vi "Translate.vi"(7 "Size":i32, 9 "direction in":enum16{"R", "D", "L", "U"}(ring), 10 "x in":i32, 11 "y in":i32) -> (1 "direction out":enum16{"R", "D", "L", "U"}(ring), 2 "x out":i32, 3 "y out":i32)   [LabVIEW 2021, in "d22.lvlib"]
uses:
  d22.lvlib
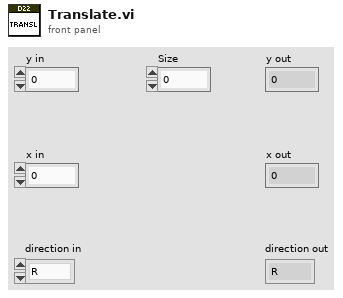
[diagram p1: front panel]
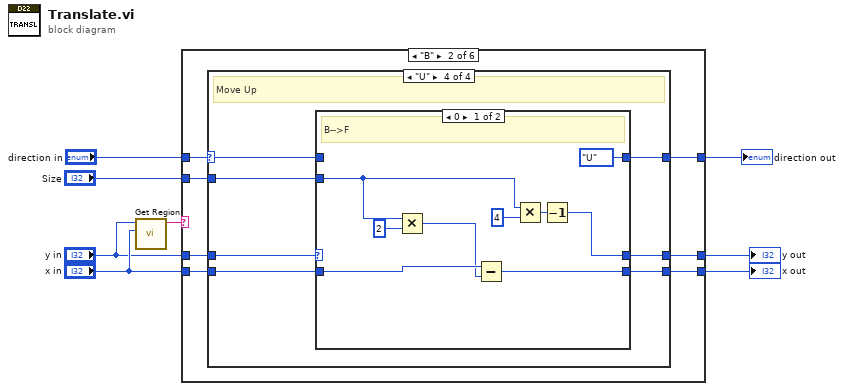
[diagram p0: block diagram]
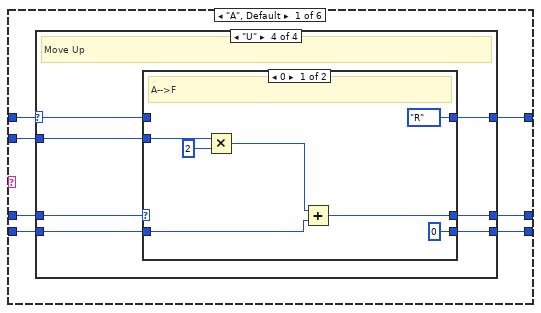
[diagram p2: hidden frame]
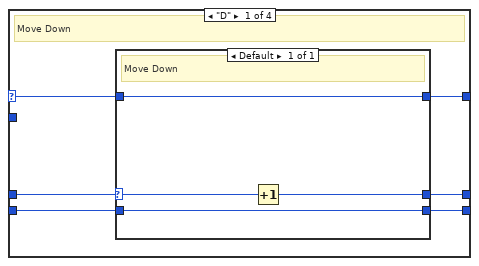
[diagram p3: hidden frame]
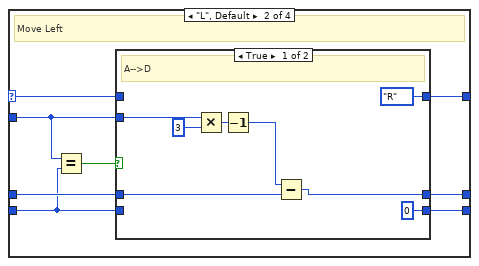
[diagram p4: hidden frame]
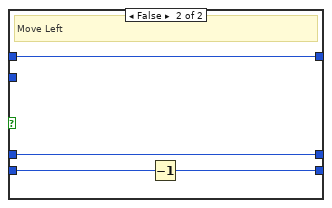
[diagram p5: hidden frame]
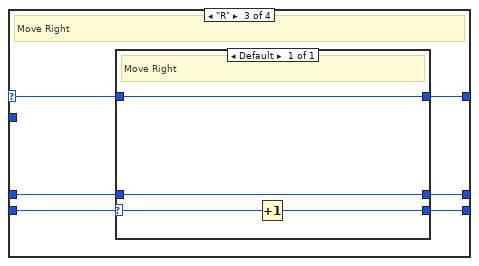
[diagram p6: hidden frame]
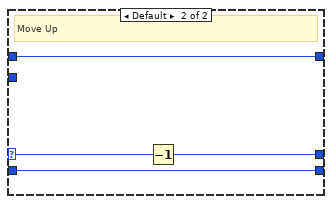
[diagram p7: hidden frame]
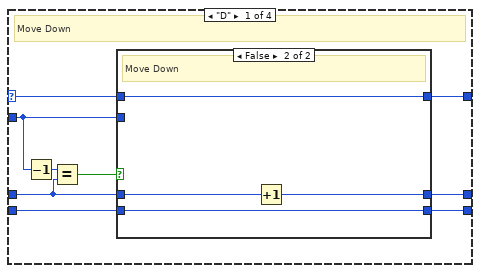
[diagram p8: hidden frame]
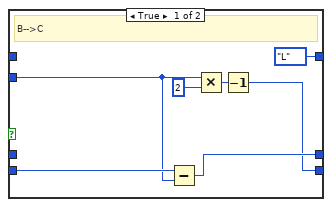
[diagram p9: hidden frame]
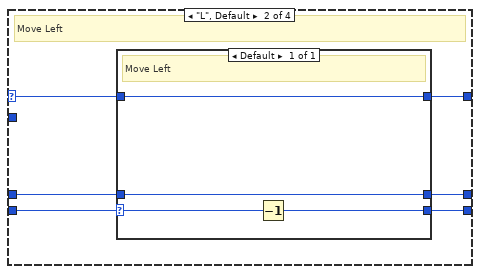
[diagram p10: hidden frame]
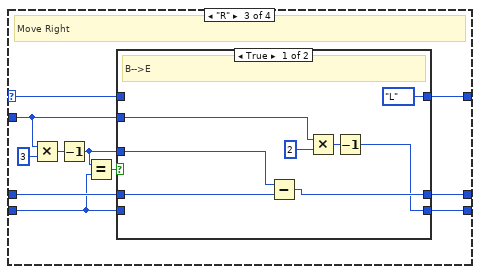
[diagram p11: hidden frame]
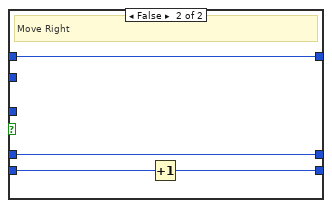
[diagram p12: hidden frame]
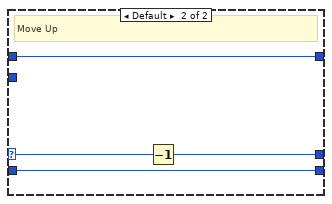
[diagram p13: hidden frame]
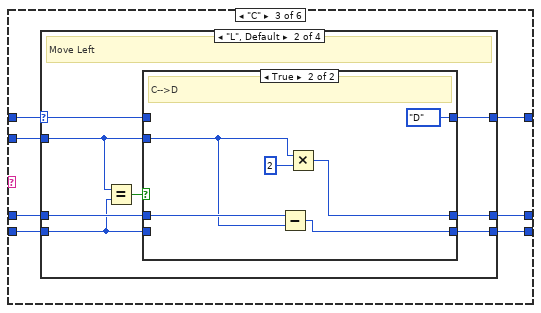
[diagram p14: hidden frame]
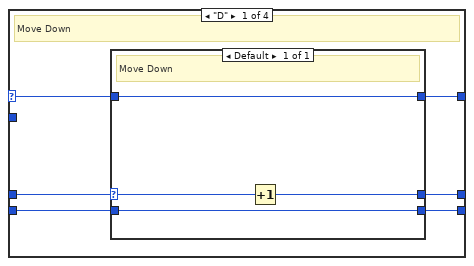
[diagram p15: hidden frame]
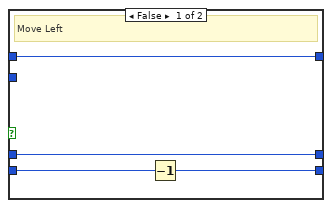
[diagram p16: hidden frame]
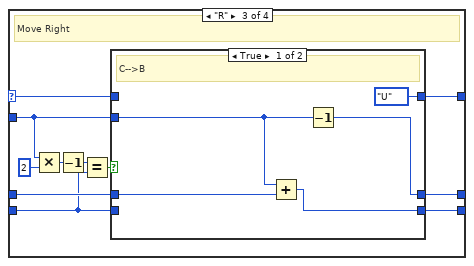
[diagram p17: hidden frame]
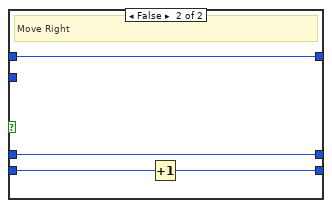
[diagram p18: hidden frame]
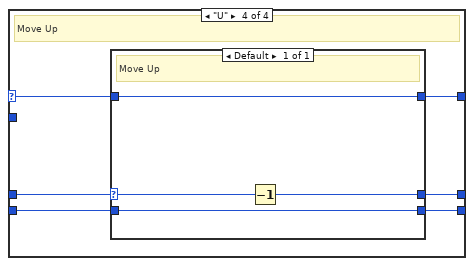
[diagram p19: hidden frame]
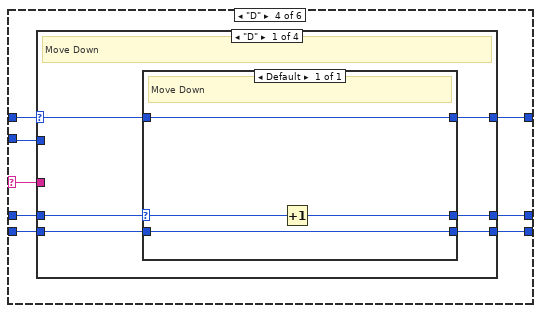
[diagram p20: hidden frame]
diagram:
  n1 = call "Get Region.vi"("x"="x in", "y"="y in") -> ("region"=w1:string)  [unwired: 9 in]
  n2 = case shown="\"B\"" w1 {
    selector: w1 -> [_ _ _ w220 _ _]
    tunnel: "y in" -> [w15 w80 w160 w226 w289 w360]
    tunnel: "x in" -> [w13 w78 w158 w224 w287 w358]
    tunnel: [w14 w79 w159 w225 w288 w359] -> w4
    tunnel: [w12 w77 w157 w223 w286 w357] -> w5
    tunnel: [w11 w76 w156 w222 w285 w356] -> w3
    tunnel: "direction in" -> [w10 w75 w155 w221 w284 w355]
    tunnel: "Size" -> [w9 w74 w154 w219 w283 w354]
    frame "A", Default {
      n3 = case shown="\"U\"" w10 {
        selector: w10 -> [w20 w33 w51 w61]
        tunnel: w15 -> [w19 w31 w50 w59]
        tunnel: [w17 w30 w47 w58] -> w14
        tunnel: w13 -> [w18 w28 w49 w62]
        tunnel: [w16 w29 w46 w57] -> w12
        tunnel: [w21 w32 w48 w60] -> w11
        tunnel: w9 -> [_ w27 _ w56]
        frame "D" {
          # "Move Down"
          n4 = case shown="Default" w19 {
            selector: w19 -> [w24]
            tunnel: w20 -> [w25]
            tunnel: [w25] -> w21
            tunnel: [w22] -> w17
            tunnel: [w23] -> w16
            tunnel: w18 -> [w23]
            frame Default {
              # "Move Down"
              n5 = Increment(x=w24) -> (x+1=w22:i32)
            }
          }
        }
        frame "L", Default {
          # "Move Left"
          n6 = Equal?(x=w27, y=w28) -> (x = y?=w26:bool)
          n7 = case shown="True" w26 {
            tunnel: w33 -> [_ w45]
            tunnel: [enum16{"R", "D", "L", "U"}."R" ("direction in") w45] -> w32
            tunnel: w31 -> [w39 w44]
            tunnel: [w38 w44] -> w30
            tunnel: [0 w42] -> w29
            tunnel: w27 -> [w34 _]
            tunnel: w28 -> [_ w43]
            frame True {
              # "A-->D"
              n8 = Multiply(x=w34, y=3) -> (x*y=w36:i32)
              n9 = Decrement(x=w36) -> (x-1=w35:i32)
              n10 = Subtract(x=w35, y=w39) -> (x-y=w38:i32)
            }
            frame False {
              # "Move Left"
              n11 = Decrement(x=w43) -> (x-1=w42:i32)
            }
          }
        }
        frame "R" {
          # "Move Right"
          n12 = case shown="Default" w49 {
            selector: w49 -> [w53]
            tunnel: w51 -> [w55]
            tunnel: [w55] -> w48
            tunnel: w50 -> [w54]
            tunnel: [w54] -> w47
            tunnel: [w52] -> w46
            frame Default {
              # "Move Right"
              n13 = Increment(x=w53) -> (x+1=w52:i32)
            }
          }
        }
        frame "U" {
          # "Move Up"
          n14 = case shown="0" w59 {
            selector: w59 -> [_ w72]
            tunnel: w61 -> [_ w73]
            tunnel: [enum16{"R", "D", "L", "U"}."R" ("direction in") w73] -> w60
            tunnel: [w67 w70] -> w58
            tunnel: [0 w71] -> w57
            tunnel: w62 -> [w63 w71]
            tunnel: w56 -> [w65 _]
            frame 0 {
              # "A-->F"
              n15 = Multiply(x=w65, y=2) -> (x*y=w64:i32)
              n16 = Add(x=w64, y=w63) -> (x+y=w67:i32)
            }
            frame Default {
              # "Move Up"
              n17 = Decrement(x=w72) -> (x-1=w70:i32)
            }
          }
        }
      }
    }
    frame "B" {
      n18 = case shown="\"U\"" w75 {
        selector: w75 -> [w88 w104 w121 w139]
        tunnel: w80 -> [w82 w106 w119 w137]
        tunnel: [w86 w102 w118 w136] -> w79
        tunnel: w78 -> [w89 w105 w111 w140]
        tunnel: [w85 w101 w117 w135] -> w77
        tunnel: [w87 w103 w120 w138] -> w76
        tunnel: w74 -> [w81 _ w114 w134]
        frame "D" {
          # "Move Down"
          n19 = Decrement(x=w81) -> (x-1=w84:i32)
          n20 = Equal?(x=w84, y=w82) -> (x = y?=w83:bool)
          n21 = case shown="False" w83 {
            tunnel: w88 -> [_ w100]
            tunnel: [enum16{"R", "D", "L", "U"}."L" ("direction in") w100] -> w87
            tunnel: [w95 w98] -> w86
            tunnel: [w90 w99] -> w85
            tunnel: w89 -> [w94 w99]
            tunnel: w82 -> [_ w97]
            tunnel: w81 -> [w91 _]
            frame True {
              # "B-->C"
              n22 = Subtract(x=w94, y=w91) -> (x-y=w95:i32)
              n23 = Multiply(x=w91, y=2) -> (x*y=w92:i32)
              n24 = Decrement(x=w92) -> (x-1=w90:i32)
            }
            frame False {
              # "Move Down"
              n25 = Increment(x=w97) -> (x+1=w98:i32)
            }
          }
        }
        frame "L", Default {
          # "Move Left"
          n26 = case shown="Default" w105 {
            selector: w105 -> [w108]
            tunnel: w104 -> [w110]
            tunnel: [w110] -> w103
            tunnel: w106 -> [w109]
            tunnel: [w109] -> w102
            tunnel: [w107] -> w101
            frame Default {
              # "Move Left"
              n27 = Decrement(x=w108) -> (x-1=w107:i32)
            }
          }
        }
        frame "R" {
          # "Move Right"
          n28 = Multiply(x=w114, y=3) -> (x*y=w115:i32)
          n29 = Decrement(x=w115) -> (x-1=w112:i32)
          n30 = Equal?(x=w112, y=w111) -> (x = y?=w113:bool)
          n31 = case shown="True" w113 {
            tunnel: w121 -> [_ w133]
            tunnel: [enum16{"R", "D", "L", "U"}."L" ("direction in") w133] -> w120
            tunnel: w119 -> [w128 w132]
            tunnel: [w127 w132] -> w118
            tunnel: [w124 w131] -> w117
            tunnel: w114 -> [w123 _]
            tunnel: w112 -> [w122 _]
            tunnel: w111 -> [_ w130]
            frame True {
              # "B-->E"
              n32 = Subtract(x=w122, y=w128) -> (x-y=w127:i32)
              n33 = Multiply(x=w123, y=2) -> (x*y=w125:i32)
              n34 = Decrement(x=w125) -> (x-1=w124:i32)
            }
            frame False {
              # "Move Right"
              n35 = Increment(x=w130) -> (x+1=w131:i32)
            }
          }
        }
        frame "U" {
          # "Move Up"
          n36 = case shown="0" w137 {
            selector: w137 -> [_ w152]
            tunnel: w139 -> [_ w153]
            tunnel: [enum16{"R", "D", "L", "U"}."U" ("direction in") w153] -> w138
            tunnel: [w141 w150] -> w136
            tunnel: [w147 w151] -> w135
            tunnel: w140 -> [w148 w151]
            tunnel: w134 -> [w142 _]
            frame 0 {
              # "B-->F"
              n37 = Multiply(x=w142, y=2) -> (x*y=w145:i32)
              n38 = Subtract(x=w148, y=w145) -> (x-y=w147:i32)
              n39 = Multiply(x=w142, y=4) -> (x*y=w143:i32)
              n40 = Decrement(x=w143) -> (x-1=w141:i32)
            }
            frame Default {
              # "Move Up"
              n41 = Decrement(x=w152) -> (x-1=w150:i32)
            }
          }
        }
      }
    }
    frame "C" {
      n42 = case shown="\"L\", Default" w155 {
        selector: w155 -> [w165 w177 w199 w213]
        tunnel: w160 -> [w163 w178 w197 w211]
        tunnel: [w162 w175 w196 w210] -> w159
        tunnel: w158 -> [w166 w172 w189 w214]
        tunnel: [w161 w174 w195 w209] -> w157
        tunnel: [w164 w176 w198 w212] -> w156
        tunnel: w154 -> [_ w173 w192 _]
        frame "D" {
          # "Move Down"
          n43 = case shown="Default" w163 {
            selector: w163 -> [w169]
            tunnel: w165 -> [w170]
            tunnel: [w170] -> w164
            tunnel: [w167] -> w162
            tunnel: [w168] -> w161
            tunnel: w166 -> [w168]
            frame Default {
              # "Move Down"
              n44 = Increment(x=w169) -> (x+1=w167:i32)
            }
          }
        }
        frame "L", Default {
          # "Move Left"
          n45 = Equal?(x=w173, y=w172) -> (x = y?=w171:bool)
          n46 = case shown="True" w171 {
            tunnel: w177 -> [w182 _]
            tunnel: [w182 enum16{"R", "D", "L", "U"}."D" ("direction in")] -> w176
            tunnel: w178 -> [w181 w187]
            tunnel: [w181 w183] -> w175
            tunnel: [w179 w186] -> w174
            tunnel: w173 -> [_ w184]
            tunnel: w172 -> [w180 _]
            frame False {
              # "Move Left"
              n47 = Decrement(x=w180) -> (x-1=w179:i32)
            }
            frame True {
              # "C-->D"
              n48 = Subtract(x=w187, y=w184) -> (x-y=w186:i32)
              n49 = Multiply(x=w184, y=2) -> (x*y=w183:i32)
            }
          }
        }
        frame "R" {
          # "Move Right"
          n50 = Multiply(x=w192, y=2) -> (x*y=w193:i32)
          n51 = Decrement(x=w193) -> (x-1=w191:i32)
          n52 = Equal?(x=w191, y=w189) -> (x = y?=w190:bool)
          n53 = case shown="True" w190 {
            tunnel: w199 -> [_ w208]
            tunnel: [enum16{"R", "D", "L", "U"}."U" ("direction in") w208] -> w198
            tunnel: w197 -> [w203 w207]
            tunnel: [w200 w207] -> w196
            tunnel: [w202 w205] -> w195
            tunnel: w192 -> [w201 _]
            tunnel: w189 -> [_ w206]
            frame True {
              # "C-->B"
              n54 = Add(x=w201, y=w203) -> (x+y=w202:i32)
              n55 = Decrement(x=w201) -> (x-1=w200:i32)
            }
            frame False {
              # "Move Right"
              n56 = Increment(x=w206) -> (x+1=w205:i32)
            }
          }
        }
        frame "U" {
          # "Move Up"
          n57 = case shown="Default" w211 {
            selector: w211 -> [w217]
            tunnel: w213 -> [w218]
            tunnel: [w218] -> w212
            tunnel: [w215] -> w210
            tunnel: [w216] -> w209
            tunnel: w214 -> [w216]
            frame Default {
              # "Move Up"
              n58 = Decrement(x=w217) -> (x-1=w215:i32)
            }
          }
        }
      }
    }
    frame "D" {
      n59 = case shown="\"D\"" w221 {
        selector: w221 -> [w231 w241 w259 w274]
        tunnel: w226 -> [w229 w243 w257 w267]
        tunnel: [w228 w239 w256 w272] -> w225
        tunnel: w224 -> [w232 w242 w260 w268]
        tunnel: [w227 w238 w255 w271] -> w223
        tunnel: [w230 w240 w258 w273] -> w222
        tunnel: w220 -> [_ _ _ _]
        tunnel: w219 -> [_ w237 _ w265]
        frame "D" {
          # "Move Down"
          n60 = case shown="Default" w229 {
            selector: w229 -> [w235]
            tunnel: w231 -> [w236]
            tunnel: [w236] -> w230
            tunnel: [w233] -> w228
            tunnel: [w234] -> w227
            tunnel: w232 -> [w234]
            frame Default {
              # "Move Down"
              n61 = Increment(x=w235) -> (x+1=w233:i32)
            }
          }
        }
        frame "L", Default {
          # "Move Left"
          n62 = case shown="0" w242 {
            selector: w242 -> [w245 _]
            tunnel: w241 -> [w247 _]
            tunnel: [w247 enum16{"R", "D", "L", "U"}."R" ("direction in")] -> w240
            tunnel: w243 -> [w246 w253]
            tunnel: [w246 w252] -> w239
            tunnel: [w244 w248] -> w238
            tunnel: w237 -> [_ w248]
            frame Default {
              # "Move Left"
              n63 = Decrement(x=w245) -> (x-1=w244:i32)
            }
            frame 0 {
              # "D-->A"
              n64 = Multiply(x=w248, y=3) -> (x*y=w250:i32)
              n65 = Decrement(x=w250) -> (x-1=w249:i32)
              n66 = Subtract(x=w249, y=w253) -> (x-y=w252:i32)
            }
          }
        }
        frame "R" {
          # "Move Right"
          n67 = case shown="Default" w260 {
            selector: w260 -> [w262]
            tunnel: w259 -> [w264]
            tunnel: [w264] -> w258
            tunnel: w257 -> [w263]
            tunnel: [w263] -> w256
            tunnel: [w261] -> w255
            frame Default {
              # "Move Right"
              n68 = Increment(x=w262) -> (x+1=w261:i32)
            }
          }
        }
        frame "U" {
          # "Move Up"
          n69 = Multiply(x=w265, y=2) -> (x*y=w269:i32)
          n70 = Equal?(x=w269, y=w267) -> (x = y?=w266:bool)
          n71 = case shown="True" w266 {
            tunnel: w274 -> [w278 _]
            tunnel: [w278 enum16{"R", "D", "L", "U"}."R" ("direction in")] -> w273
            tunnel: [w275 w281] -> w272
            tunnel: [w276 w280] -> w271
            tunnel: w268 -> [w276 w279]
            tunnel: w267 -> [w277 _]
            tunnel: w265 -> [_ w280]
            frame False {
              # "Move Up"
              n72 = Decrement(x=w277) -> (x-1=w275:i32)
            }
            frame True {
              # "D-->C"
              n73 = Add(x=w280, y=w279) -> (x+y=w281:i32)
            }
          }
        }
      }
    }
    frame "E" {
      n74 = case shown="\"R\"" w284 {
        selector: w284 -> [w299 w315 w332 w348]
        tunnel: w289 -> [w292 w317 w330 w346]
        tunnel: [w297 w313 w329 w345] -> w288
        tunnel: w287 -> [w300 w316 w324 w349]
        tunnel: [w296 w312 w328 w344] -> w286
        tunnel: [w298 w314 w331 w347] -> w285
        tunnel: w283 -> [w290 _ w322 _]
        frame "D" {
          # "Move Down"
          n75 = Multiply(x=w290, y=3) -> (x*y=w294:i32)
          n76 = Decrement(x=w294) -> (x-1=w293:i32)
          n77 = Equal?(x=w293, y=w292) -> (x = y?=w291:bool)
          n78 = case shown="True" w291 {
            tunnel: w299 -> [w304 _]
            tunnel: [w304 enum16{"R", "D", "L", "U"}."L" ("direction in")] -> w298
            tunnel: [w301 w309] -> w297
            tunnel: [w302 w305] -> w296
            tunnel: w300 -> [w302 w310]
            tunnel: w292 -> [w303 _]
            tunnel: w290 -> [_ w306]
            frame False {
              # "Move Down"
              n79 = Increment(x=w303) -> (x+1=w301:i32)
            }
            frame True {
              # "E-->F"
              n80 = Multiply(x=w306, y=2) -> (x*y=w307:i32)
              n81 = Add(x=w307, y=w310) -> (x+y=w309:i32)
              n82 = Decrement(x=w306) -> (x-1=w305:i32)
            }
          }
        }
        frame "L", Default {
          # "Move Left"
          n83 = case shown="Default" w316 {
            selector: w316 -> [w319]
            tunnel: w315 -> [w321]
            tunnel: [w321] -> w314
            tunnel: w317 -> [w320]
            tunnel: [w320] -> w313
            tunnel: [w318] -> w312
            frame Default {
              # "Move Left"
              n84 = Decrement(x=w319) -> (x-1=w318:i32)
            }
          }
        }
        frame "R" {
          # "Move Right"
          n85 = Multiply(x=w322, y=2) -> (x*y=w326:i32)
          n86 = Decrement(x=w326) -> (x-1=w325:i32)
          n87 = Equal?(x=w325, y=w324) -> (x = y?=w323:bool)
          n88 = case shown="True" w323 {
            tunnel: w332 -> [w336 _]
            tunnel: [w336 enum16{"R", "D", "L", "U"}."L" ("direction in")] -> w331
            tunnel: w330 -> [w335 w343]
            tunnel: [w335 w342] -> w329
            tunnel: [w333 w337] -> w328
            tunnel: w324 -> [w334 _]
            tunnel: w322 -> [_ w338]
            frame False {
              # "Move Right"
              n89 = Increment(x=w334) -> (x+1=w333:i32)
            }
            frame True {
              # "E-->B"
              n90 = Multiply(x=w338, y=3) -> (x*y=w339:i32)
              n91 = Decrement(x=w339) -> (x-1=w337:i32)
              n92 = Subtract(x=w337, y=w343) -> (x-y=w342:i32)
            }
          }
        }
        frame "U" {
          # "Move Up"
          n93 = case shown="Default" w346 {
            selector: w346 -> [w352]
            tunnel: w348 -> [w353]
            tunnel: [w353] -> w347
            tunnel: [w350] -> w345
            tunnel: [w351] -> w344
            tunnel: w349 -> [w351]
            frame Default {
              # "Move Up"
              n94 = Decrement(x=w352) -> (x-1=w350:i32)
            }
          }
        }
      }
    }
    frame "F" {
      n95 = case shown="\"D\"" w355 {
        selector: w355 -> [w370 w387 w409 w427]
        tunnel: w360 -> [w363 w389 w407 w425]
        tunnel: [w368 w385 w406 w424] -> w359
        tunnel: w358 -> [w371 w388 w403 w428]
        tunnel: [w367 w384 w405 w423] -> w357
        tunnel: [w369 w386 w408 w426] -> w356
        tunnel: w354 -> [w361 w383 w401 _]
        frame "D" {
          # "Move Down"
          n96 = Multiply(x=w361, y=4) -> (x*y=w365:i32)
          n97 = Decrement(x=w365) -> (x-1=w364:i32)
          n98 = Equal?(x=w364, y=w363) -> (x = y?=w362:bool)
          n99 = case shown="True" w362 {
            tunnel: w370 -> [w375 _]
            tunnel: [w375 enum16{"R", "D", "L", "U"}."D" ("direction in")] -> w369
            tunnel: [w372 0 ("x in")] -> w368
            tunnel: [w373 w379] -> w367
            tunnel: w371 -> [w373 w381]
            tunnel: w363 -> [w374 _]
            tunnel: w361 -> [_ w377]
            frame False {
              # "Move Down"
              n100 = Increment(x=w374) -> (x+1=w372:i32)
            }
            frame True {
              # "F-->B"
              n101 = Multiply(x=w377, y=2) -> (x*y=w376:i32)
              n102 = Add(x=w376, y=w381) -> (x+y=w379:i32)
            }
          }
        }
        frame "L", Default {
          # "Move Left"
          n103 = case shown="0" w388 {
            selector: w388 -> [w391 _]
            tunnel: w387 -> [w393 _]
            tunnel: [w393 enum16{"R", "D", "L", "U"}."D" ("direction in")] -> w386
            tunnel: w389 -> [w392 w398]
            tunnel: [w392 0 ("y in")] -> w385
            tunnel: [w390 w397] -> w384
            tunnel: w383 -> [_ w395]
            frame Default {
              # "Move Left"
              n104 = Decrement(x=w391) -> (x-1=w390:i32)
            }
            frame 0 {
              # "F-->A"
              n105 = Multiply(x=w395, y=2) -> (x*y=w394:i32)
              n106 = Subtract(x=w398, y=w394) -> (x-y=w397:i32)
            }
          }
        }
        frame "R" {
          # "Move Right"
          n107 = Decrement(x=w401) -> (x-1=w404:i32)
          n108 = Equal?(x=w404, y=w403) -> (x = y?=w402:bool)
          n109 = case shown="True" w402 {
            tunnel: w409 -> [w413 _]
            tunnel: [w413 enum16{"R", "D", "L", "U"}."U" ("direction in")] -> w408
            tunnel: w407 -> [w412 w422]
            tunnel: [w412 w414] -> w406
            tunnel: [w410 w420] -> w405
            tunnel: w403 -> [w411 _]
            tunnel: w401 -> [_ w415]
            frame False {
              # "Move Right"
              n110 = Increment(x=w411) -> (x+1=w410:i32)
            }
            frame True {
              # "F-->E"
              n111 = Multiply(x=w415, y=2) -> (x*y=w418:i32)
              n112 = Subtract(x=w422, y=w418) -> (x-y=w420:i32)
              n113 = Multiply(x=w415, y=3) -> (x*y=w416:i32)
              n114 = Decrement(x=w416) -> (x-1=w414:i32)
            }
          }
        }
        frame "U" {
          # "Move Up"
          n115 = case shown="Default" w425 {
            selector: w425 -> [w431]
            tunnel: w427 -> [w432]
            tunnel: [w432] -> w426
            tunnel: [w429] -> w424
            tunnel: [w430] -> w423
            tunnel: w428 -> [w430]
            frame Default {
              # "Move Up"
              n116 = Decrement(x=w431) -> (x-1=w429:i32)
            }
          }
        }
      }
    }
  }
  "x out" <- w5
  "y out" <- w4
  "direction out" <- w3
